vi "GT Get Remainder Seg Num.vi"(7 "fifo":i16, 8 "error in (no error)":errorcluster caption="错误输入（无错误）", 9 "pSegment":i32, 10 "crd":i16, 11 "cardNum":i16) -> (0 "error out":errorcluster caption="错误输出", 1 "pSegment out":i32, 3 "function return":i16)   [LabVIEW 2020, in "gts.lvlib"]
doc: "GT_API GT_GetRemainderSegNum(short cardNum,short crd,long *pSegment,short fifo=0);"
uses:
  gts.lvlib
  dll/32bit/multi_card/gts.dll
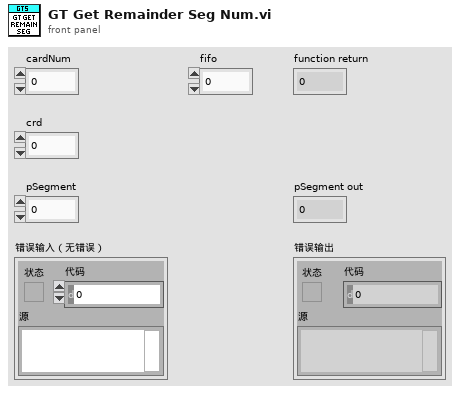
[diagram p1: front panel]
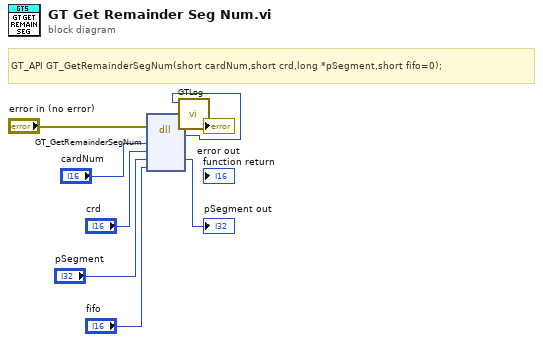
[diagram p0: block diagram]
diagram:
  # "GT_API GT_GetRemainderSegNum(short cardNum,short crd,long *pSegment,short fifo=0);"
  n1 = dll-call lib="C:/1228/dll/32bit/multi_card/gts.dll" fn="GT_GetRemainderSegNum"(error in="error in (no error)", "cardNum"="cardNum", "crd"="crd", "pSegment"="pSegment", "fifo"="fifo") -> (error out=w3:errorcluster, w1:i16, "pSegment"=→"pSegment out":i32)  [unwired: 5 in, 1 out]
  n2 = call "GTLog.vi"("error in (no error)"=w3, "Numeric"=w1) -> ("error out"=→"error out":errorcluster)  [unwired: 9 in]
